vi "subwhatever.vi"() -> ()   [LabVIEW 2010]
panel:
  in  "Your initials 3":string
  in  "parent class":path
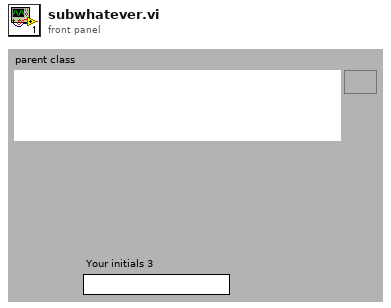
[diagram p1: front panel]
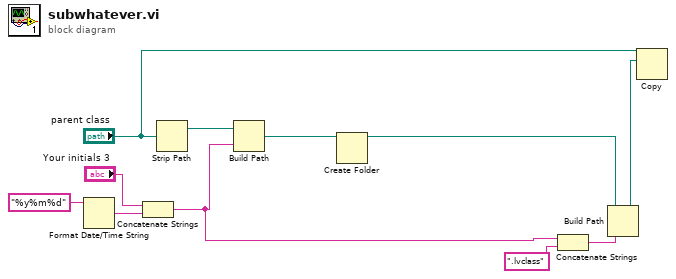
[diagram p0: block diagram]
diagram:
  n1 = Format Date/Time String(time format string (%c)="%y%m%d") -> (date/time string=w8:string)  [unwired: 2 in]
  n2 = Concatenate Strings("Your initials 3", w8) -> (w4:string)
  n3 = Strip Path(path="parent class") -> (stripped path=w7:path)  [unwired: 1 out]
  n4 = Build Path(base path=w7, name or relative path=w4) -> (appended path=w11:path)
  n5 = Create Folder(path (use dialog)=w11) -> (created path=w1:path)  [unwired: 2 in, 2 out]
  n6 = Concatenate Strings(w4, ".lvclass" ("string")) -> (w3:string)
  n7 = Build Path(base path=w1, name or relative path=w3) -> (appended path=w5:path)
  n8 = Copy(10:w5, 11:"parent class") -> ()  [unwired: 3 in, 3 out]
